vi "Write Server address.vi"(8 "error in (no error)":errorcluster, 10 "Server address":string="192.168.1.100", 11 "RP Instrument in":refnum<class "RP Instrument.lvclass">) -> (0 "error out":errorcluster, 3 "RP Instrument out":refnum<class "RP Instrument.lvclass">)   [LabVIEW 2019, in "RP Instrument.lvclass"]
uses:
  RP Instrument.lvclass
  RP Instrument.lvclass/RP Instrument.ctl
  RP Communicator/RP Communicator.lvclass
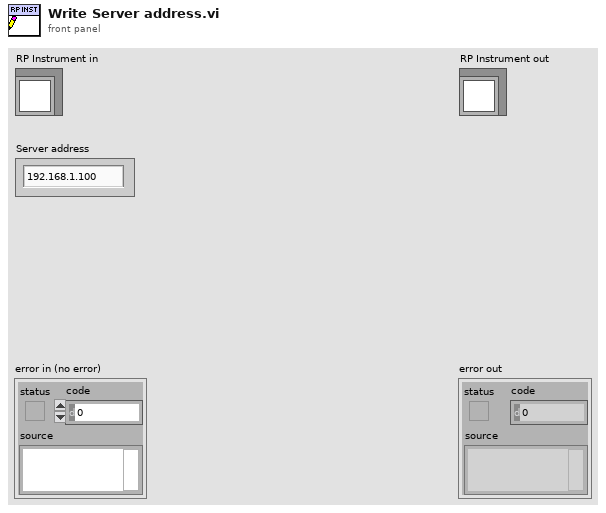
[diagram p1: front panel]
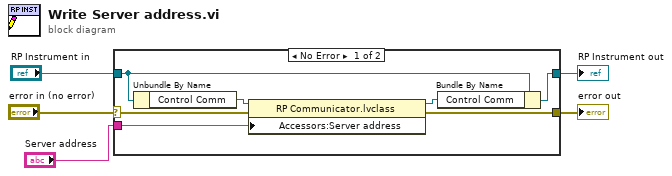
[diagram p0: block diagram]
diagram:
  n1 = case shown="No Error" "error in (no error)" {
    selector: "error in (no error)" -> [w6 w13]
    tunnel: [w7 w13] -> w4
    tunnel: [w12 w14] -> w2
    tunnel: "RP Instrument in" -> [w9 w14]
    tunnel: "Server address" -> [w10 _]
    frame No Error {
      n2 = Unbundle By Name(w9) -> ("Control Comm"=w11:refnum<class "RP Communicator.lvclass">)
      n3 = property class="RP Communicator.lvclass"(reference=w11, error in=w6, "Accessors:Server address"=w10) -> (reference out=w8:refnum<class "RP Communicator.lvclass">, error out=w7:errorcluster)
      n4 = Bundle By Name(cluster=w9, "Control Comm"=w8) -> (w12:refnum<class "RP Instrument.lvclass">)
    }
    frame Error {
    }
  }
  "error out" <- w4
  "RP Instrument out" <- w2
